vi "Render Partial.vi"(8 "Error In":errorcluster, 10 "Partial":refnum<class "Partial.lvclass">, 11 "Renderer In":refnum<class "Renderer.lvclass">) -> (0 "Error Out":errorcluster, 2 "Output":string, 3 "Renderer Out":refnum<class "Renderer.lvclass">)   [LabVIEW 2018, in "Toolkit.lvlib" / "Renderer.lvclass"]
uses:
  Renderer.lvclass
  Nodes/Partial/Partial.lvclass
  Nodes/Partial/Partial.lvclass/Partial.ctl
  Renderer.lvclass/Renderer.ctl
  Readers/String/String.lvclass
  D:/Users/cfield/Code/Field R&D Services/Labstache/src/Toolkit/Low-Level/Readers/Reader/Reader.lvclass
  Loaders/Loader/Loader.lvclass
  Lexer/Lexer.lvclass
  Parser/Parser.lvclass
  Nodes/Root/Root.lvclass
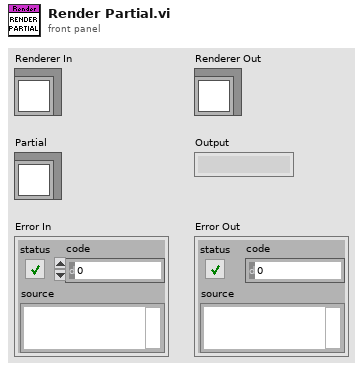
[diagram p1: front panel]
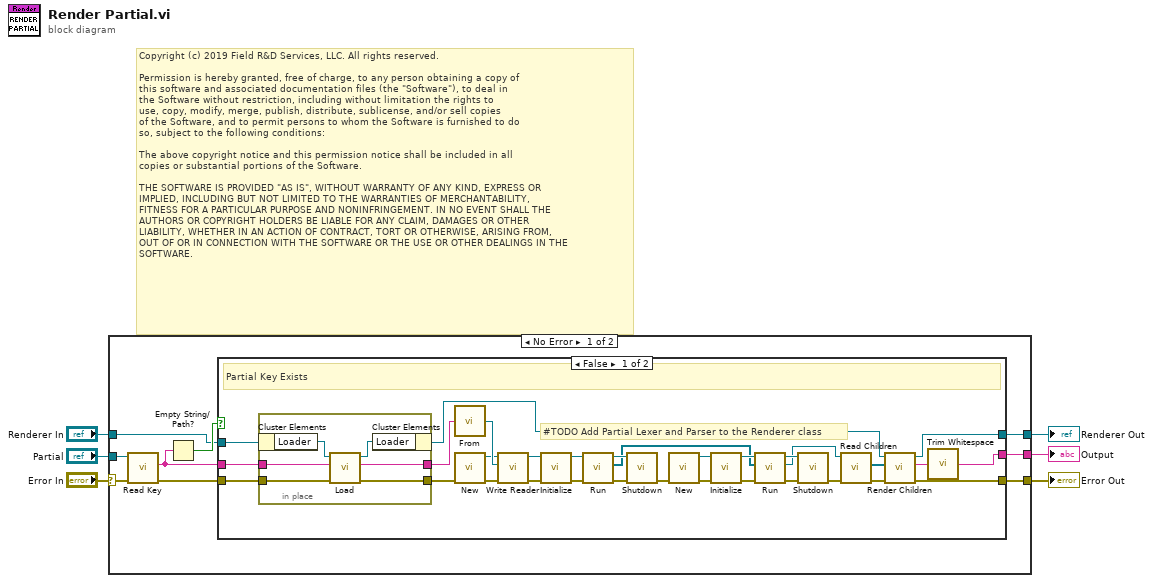
[diagram p0: block diagram]
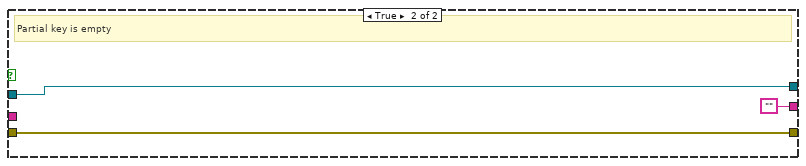
[diagram p2: hidden frame]
diagram:
  # "Copyright (c) 2019 Field R&D Services, LLC. All rights reserved.\n\nPermission is hereby granted, free of charge, to any person obtaining a copy of\nthis software and associated documentation files (the \"Software\"), to deal in\nthe Software without restriction, including without limitation the rights to\nuse, copy, modify, merge, publish, distribute, sublicense, and/or sell copies\nof the Software, and to permit persons to whom the Software is furnished to do\nso, subject to the following conditions:\n\nThe above copyright notice and this permission notice shall be included in all\ncopies or substantial portions of the Software.\n\nTHE SOFTWARE IS PROVIDED \"AS IS\", WITHOUT WARRANTY OF ANY KIND, EXPRESS OR\nIMPLIED, INCLUDING BUT NOT LIMITED TO THE WARRANTIES OF MERCHANTABILITY,\nFITNESS FOR A PARTICULAR PURPOSE AND NONINFRINGEMENT. IN NO EVENT SHALL THE\nAUTHORS OR COPYRIGHT HOLDERS BE LIABLE FOR ANY CLAIM, DAMAGES OR OTHER\nLIABILITY, WHETHER IN AN ACTION OF CONTRACT, TORT OR OTHERWISE, ARISING FROM,\nOUT OF OR IN CONNECTION WITH THE SOFTWARE OR THE USE OR OTHER DEALINGS IN THE\nSOFTWARE."
  n1 = case shown="No Error" "Error In" {
    selector: "Error In" -> [w12 w56]
    tunnel: "Partial" -> [w10 _]
    tunnel: [w9 w56] -> w5
    tunnel: [w8 w57] -> w1
    tunnel: "Renderer In" -> [w11 w57]
    tunnel: [w7 _] -> w3
    frame No Error {
      n2 = call "Read Key.vi"("Error In"=w12, "Partial In"=w10) -> ("Error Out"=w14:errorcluster, "Key"=w13:string)  [unwired: 7 in, 1 out]
      n3 = Empty String/Path?(string/path=w13) -> (empty?=w15:bool)
      n4 = case shown="False" w15 {
        tunnel: [w39 ""] -> w7
        tunnel: w11 -> [w38 w54]
        tunnel: [w43 w54] -> w8
        tunnel: w14 -> [w45 w53]
        tunnel: [w42 w53] -> w9
        tunnel: w13 -> [w46 _]
        frame False {
          # "#TODO Add Partial Lexer and Parser to the Renderer class"
          # "Partial Key Exists"
          n5 = in-place {
            in-place-border: w46 -> [w52]
            in-place-border: w45 -> [w51]
            in-place-border: [w50] -> w36
            in-place-border: [w49] -> w35
            n6 = in-place-cluster #1(w38) -> ("Loader"=w48:refnum<class "Loader.lvclass">)
            n7 = call-dynamic "Load.vi"("Error In"=w51, "Key"=w52, "Loader In"=w48) -> ("Error Out"=w50:errorcluster, "Template"=w49:string, "Loader Out"=w47:refnum<class "Loader.lvclass">)  [unwired: 6 in]
            n8 = in-place-cluster #1("Loader"=w47) -> (w37:refnum<class "Renderer.lvclass">)
          }
          n9 = call "From.vi"("Value"=w35) -> ("String"=w34:refnum<class "String.lvclass">)
          n10 = call "New.vi"("Error In"=w36) -> ("Error Out"=w32:errorcluster, "Lexer"=w33:refnum<class "Lexer.lvclass">)  [unwired: 9 in]
          n11 = call-dynamic "Write Reader.vi"("Error In"=w32, "Reader"=w34, "Lexer In"=w33) -> ("Error Out"=w30:errorcluster, "Lexer Out"=w31:refnum<class "Lexer.lvclass">)  [unwired: 7 in]
          n12 = call-dynamic "Initialize.vi"("Error In"=w30, "Lexer In"=w31) -> ("Error Out"=w28:errorcluster, "Lexer Out"=w29:refnum<class "Lexer.lvclass">)  [unwired: 8 in]
          n13 = call-dynamic "Run.vi"("Error In"=w28, "Lexer In"=w29) -> ("Error Out"=w26:errorcluster, "Tokens"=w16:refnum<class "Token.lvclass">[], "Lexer Out"=w27:refnum<class "Lexer.lvclass">)  [unwired: 7 in]
          n14 = call-dynamic "Shutdown.vi"("Error In"=w26, "Lexer In"=w27) -> ("Error Out"=w25:errorcluster)  [unwired: 8 in, 1 out]
          n15 = call "New.vi"("Error In"=w25) -> ("Error Out"=w23:errorcluster, "Parser"=w24:refnum<class "Parser.lvclass">)  [unwired: 9 in]
          n16 = call-dynamic "Initialize.vi"("Error In"=w23, "Parser In"=w24) -> ("Error Out"=w21:errorcluster, "Parser Out"=w22:refnum<class "Parser.lvclass">)  [unwired: 8 in]
          n17 = call-dynamic "Run.vi"("Error In"=w21, "Tokens"=w16, "Parser In"=w22) -> ("Error Out"=w19:errorcluster, "Abstract Syntax Tree"=w17:refnum<class "Root.lvclass">, "Parser Out"=w20:refnum<class "Parser.lvclass">)  [unwired: 6 in]
          n18 = call-dynamic "Shutdown.vi"("Error In"=w19, "Parser In"=w20) -> ("Error Out"=w18:errorcluster)  [unwired: 8 in, 1 out]
          n19 = call-dynamic "Read Children.vi"("Error In"=w18, "Non-Terminal In"=w17) -> ("Error Out"=w41:errorcluster, "Children"=w44:refnum<class "Node.lvclass">[])  [unwired: 7 in, 1 out]
          n20 = call "Render Children.vi"("Error In"=w41, "Children"=w44, "Renderer In"=w37) -> ("Error Out"=w42:errorcluster, "Output"=w40:string, "Renderer Out"=w43:refnum<class "Renderer.lvclass">)  [unwired: 6 in]
          n21 = call <vilib>:"Trim Whitespace.vi"("string"=w40) -> ("trimmed string"=w39:string)  [unwired: 1 in]
        }
        frame True {
          # "Partial key is empty"
        }
      }
    }
    frame Error {
    }
  }
  "Error Out" <- w5
  "Output" <- w3
  "Renderer Out" <- w1
